vi "LS330_Read_Ramp.vi"(8 "error in":errorcluster, 10 "Heater":string(combo)="1", 11 "VISA resource name":refnum<visa-resource-name>) -> (0 "error out":errorcluster, 2 "Ramp Value":dbl format="%#_6f", 3 "VISA resource name out":refnum<visa-resource-name>, 4 "Ramp Mode On/Off":bool, 6 "Ramp Busy On/Off":bool)   [LabVIEW 2021]
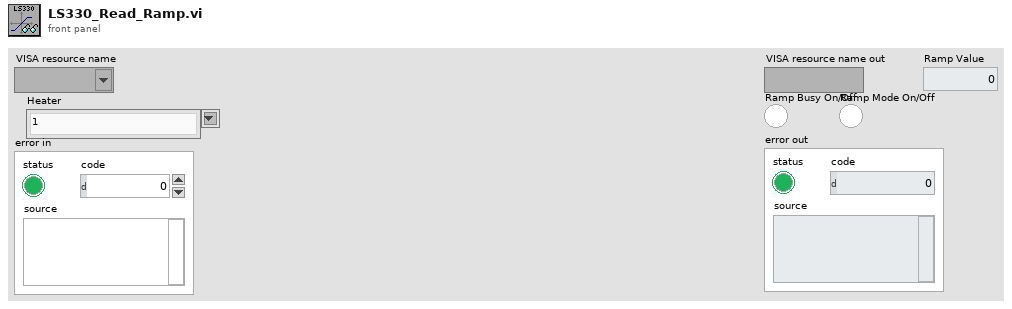
[diagram p1: front panel]
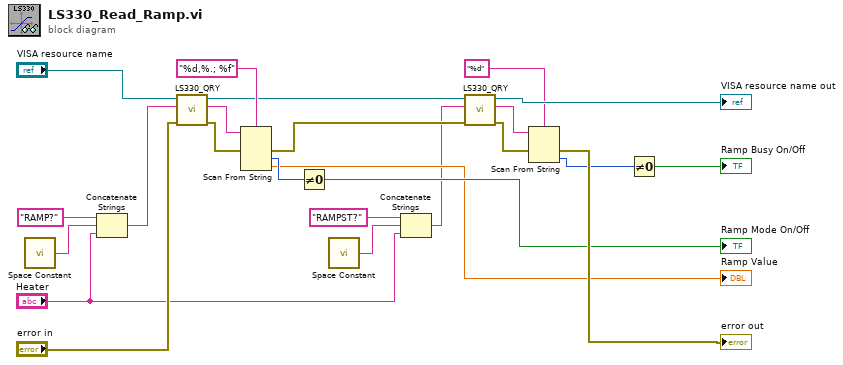
[diagram p0: block diagram]
diagram:
  n1 = call <vilib>:"Space Constant.vi"() -> ("String"=w22:string)
  n2 = Concatenate Strings("RAMP?" ("string"), w22, "Heater") -> (w21:string)
  n3 = call "LS330_QRY.vi"("error in"="error in", "CMD"=w21, "VISA resource name"="VISA resource name") -> ("error out"=w13:errorcluster, "OUT"=w14:string, "VISA resource name out"=w12:refnum<visa-resource-name>)  [unwired: 5 in, 1 out]
  n4 = Scan From String(format string="%d,%.; %f", input string=w14, error in=w13) -> (error out=w11:errorcluster, output 1=w18:i32, output 2=→"Ramp Value":dbl)  [unwired: 3 in, 2 out]
  n5 = Not Equal To 0?(x=w18) -> (x != 0?=→"Ramp Mode On/Off":bool)
  n6 = call <vilib>:"Space Constant.vi"() -> ("String"=w9:string)
  n7 = Concatenate Strings("RAMPST?" ("string"), w9, "Heater") -> (w7:string)
  n8 = call "LS330_QRY.vi"("error in"=w11, "CMD"=w7, "VISA resource name"=w12) -> ("error out"=w3:errorcluster, "OUT"=w6:string, "VISA resource name out"=→"VISA resource name out":refnum<visa-resource-name>)  [unwired: 5 in, 1 out]
  n9 = Scan From String(format string="%d", input string=w6, error in=w3) -> (error out=→"error out":errorcluster, output 1=w2:i32)  [unwired: 2 in, 2 out]
  n10 = Not Equal To 0?(x=w2) -> (x != 0?=→"Ramp Busy On/Off":bool)
